vi "DAQ.Start.Override.vi"(8 "error in (no error)":errorcluster, 11 "DAQmx in":refnum<class "DAQmx.lvclass">) -> (0 "error out":errorcluster, 3 "DAQmx out":refnum<class "DAQmx.lvclass">)   [LabVIEW 2016, in "DAQmx.lvclass"]
uses:
  DAQmx.lvclass
  DAQmx.lvclass/DAQmx.ctl
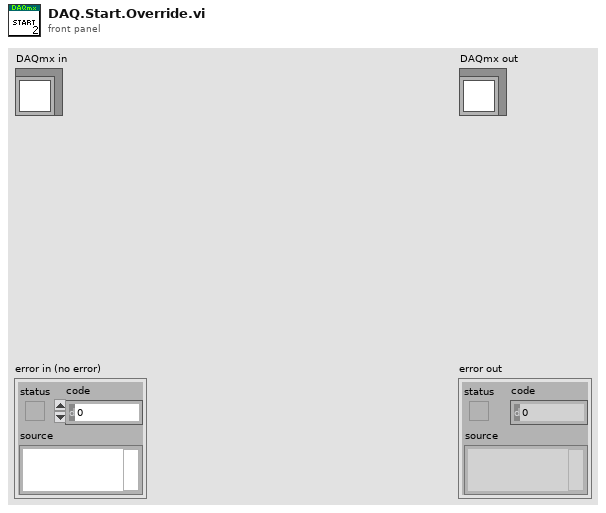
[diagram p1: front panel]
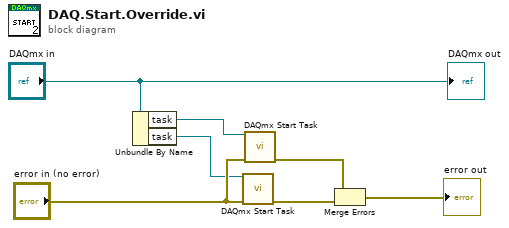
[diagram p0: block diagram]
diagram:
  n1 = Unbundle By Name("DAQmx in") -> ("task"=w7:refnum<k21>, "task"=w1:refnum<k21>)
  n2 = call <vilib>:"DAQmx Start Task.vi"("task/channels in"=w1, "error in"="error in (no error)") -> ("error out"=w4:errorcluster)  [unwired: 12 in, 1 out]
  n3 = call <vilib>:"DAQmx Start Task.vi"("task/channels in"=w7, "error in"="error in (no error)") -> ("error out"=w5:errorcluster)  [unwired: 12 in, 1 out]
  n4 = Merge Errors(w5, w4) -> (→"error out":errorcluster)
  "DAQmx out" <- "DAQmx in"
